vi "Get All Joint Positions.vi"(6 "Coordinate Space":enum16{"Color Space", "Depth Space"}(ring), 8 "error in (no error)":errorcluster, 9 "Body Index":i32) -> (0 "error out":errorcluster)   [LabVIEW 2014, in "LVH-KinectOne.lvlib"]
uses:
  LVH-KinectOne.lvlib
  Type Defs/JointType.ctl
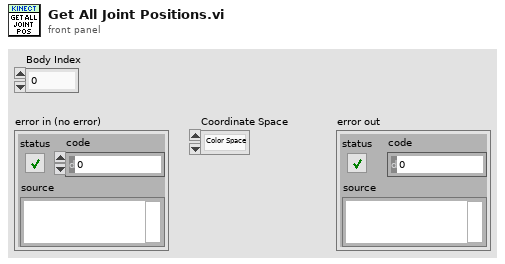
[diagram p1: front panel]
types:
  T1 = enum16{"Get Joint Position", "Initialize", "Set Joint Position"}
  T2 = typedef "LVH-KinectOne.lvlib/JointType.ctl" = i32
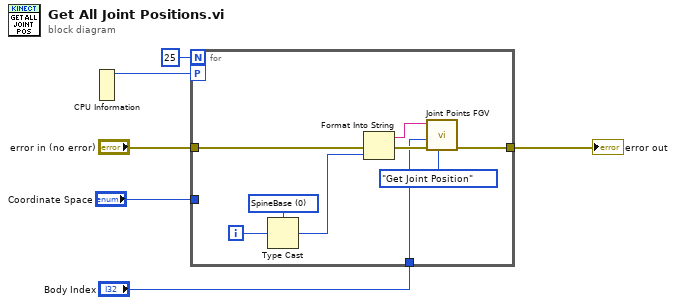
[diagram p0: block diagram]
diagram:
  n1 = CPU Information() -> (4:w1:i32)  [unwired: 3 out]
  n2 = for {
    N: 25 -> [_]
    tunnel: "Coordinate Space" -> [_]
    tunnel: "error in (no error)" -> [w7]
    tunnel: [w10] -> w3
    workers-P: w1 -> [_]
    tunnel: "Body Index" -> [w8]
    i -> [w15]
    w14 = T2 0 items=["SpineBase", "SpineMid", "Neck", "Head", "ShoulderLeft", "ElbowLeft", "WristLeft", "HandLeft", "ShoulderRight", "ElbowRight", "WristRight", "HandRight", "HipLeft", "KneeLeft", "AnkleLeft", "FootLeft", "HipRight", "KneeRight", "AnkleRight", "FootRight", "SpineShoulder", "HandTipLeft", "ThumbLeft", "HandTipRight", "ThumbRight"] ("JointType")
    n3 = Type Cast(type=w14, x=w15) -> (*(type *) &x=w11:T2)
    n4 = Format Into String(error in=w7, w11) -> (resulting string=w13:string, error out=w12:errorcluster)  [unwired: 2 in]
    n5 = call "Joint Points FGV.vi"("Command"=T1."Get Joint Position", "error in (no error)"=w12, "Body Index"=w8, "name"=w13) -> ("error out"=w10:errorcluster)  [unwired: 6 in, 1 out]
  }
  "error out" <- w3
